vi "PJT_02.vi"() -> ()   [LabVIEW 2019]
panel:
  in  "불리언 2":bool
  out "Table":string[][](table) caption="테이블"
  out "불리언":bool
  in  "정지":bool
  out "웨이브폼 그래프":dynamicdata(graph)
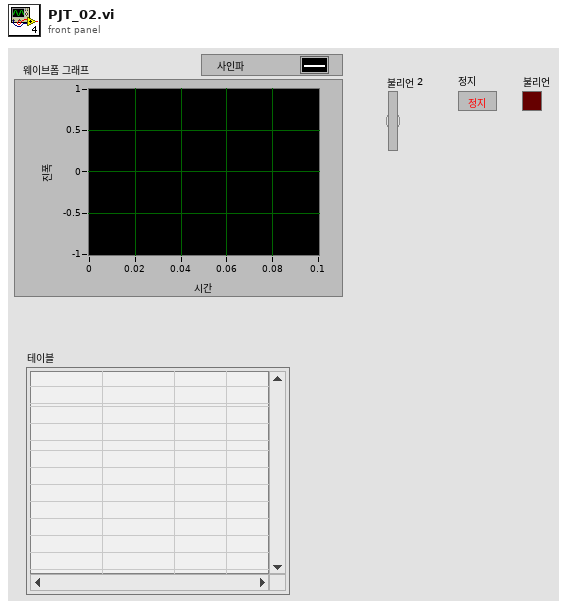
[diagram p1: front panel]
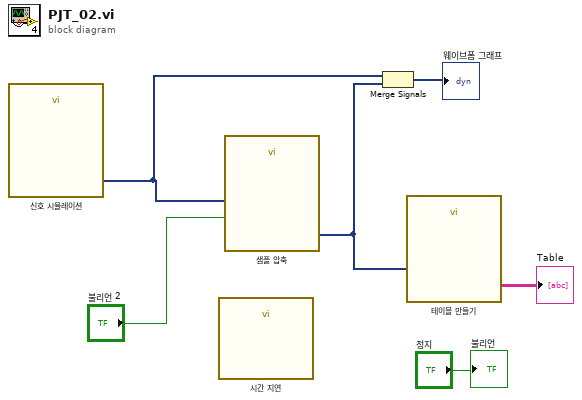
[diagram p0: block diagram]
diagram:
  n1 = call "신호 시뮬레이션"() -> ("사인파"=w3:dynamicdata)  [unwired: 14 in, 1 out]
  n2 = call "시간 지연"() -> ()  [unwired: 11 in, 1 out]
  n3 = call "샘플 압축"("Enable"="불리언 2", "Signals"=w3) -> ("Mean"=w1:dynamicdata)  [unwired: 7 in, 2 out]
  n4 = Merge Signals(w3, w1) -> (→"웨이브폼 그래프":dynamicdata)
  n5 = call "테이블 만들기"("Signals"=w1) -> ("Table"=→"Table":string[][])  [unwired: 4 in, 6 out]
  "불리언" <- "정지"
